vi "start.vi"(8 "error in (no error)":errorcluster, 11 "DAQmx_pulse_out in":refnum<class "DAQmx_DO.lvclass">) -> (0 "error out":errorcluster, 3 "DAQmx_pulse_out out":refnum<class "DAQmx_DO.lvclass">)   [LabVIEW 2013, in "DAQmx_DO.lvclass"]
uses:
  DAQmx_DO.lvclass
  DAQmx_DO.lvclass/DAQmx_DO.ctl
  Globals.vi
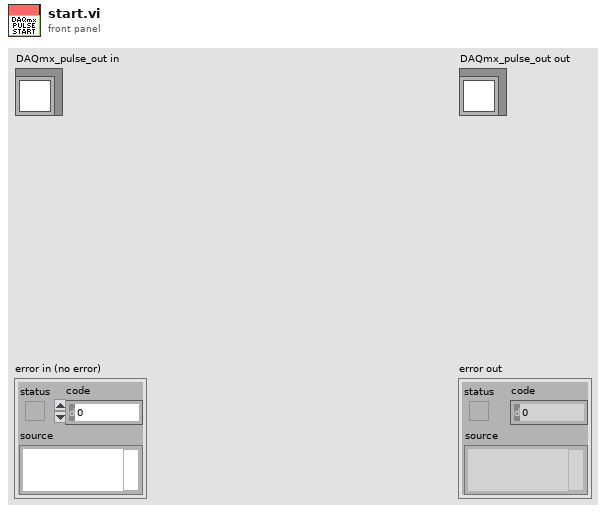
[diagram p1: front panel]
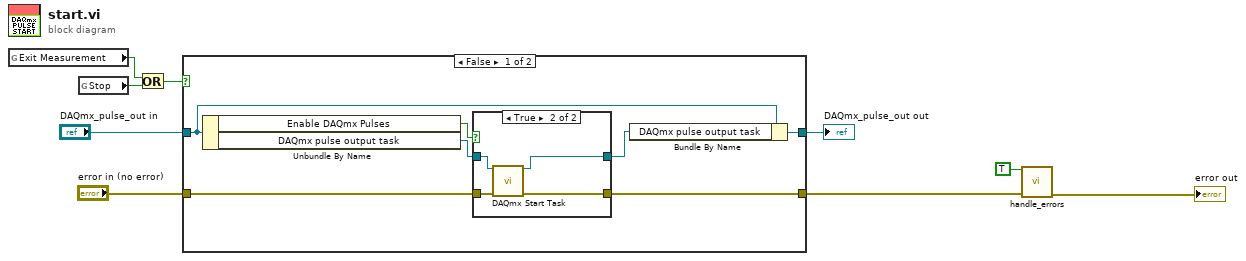
[diagram p0: block diagram]
diagram:
  n1 = global read "Globals.vi" "Exit Measurement"() -> (w6:bool)
  n2 = global read "Globals.vi" "Stop"() -> (w7:bool)
  n3 = Or(x=w6, y=w7) -> (x .or. y?=w5:bool)
  n4 = case shown="False" w5 {
    tunnel: [w11 w23] -> w2
    tunnel: [w13 w24] -> w8
    tunnel: "DAQmx_pulse_out in" -> [w14 w24]
    tunnel: "error in (no error)" -> [w10 w23]
    frame False {
      n5 = Unbundle By Name(w14) -> ("Enable DAQmx Pulses"=w16:bool, "DAQmx pulse output task"=w15:refnum<k21>)
      n6 = case shown="True" w16 {
        tunnel: w10 -> [w18 w22]
        tunnel: w15 -> [w17 w21]
        tunnel: [w18 w19] -> w11
        tunnel: [w17 w20] -> w12
        frame False {
        }
        frame True {
          n7 = call <vilib>:"DAQmx Start Task.vi"("task/channels in"=w21, "error in"=w22) -> ("task out"=w20:refnum<k21>, "error out"=w19:errorcluster)  [unwired: 12 in]
        }
      }
      n8 = Bundle By Name(cluster=w14, "DAQmx pulse output task"=w12) -> (w13:refnum<class "DAQmx_DO.lvclass">)
    }
    frame True {
    }
  }
  "DAQmx_pulse_out out" <- w8
  n9 = call "handle_errors.vi"("Exit Operation"=TRUE ("Exit Measurement"), "error in (no error)"=w2) -> ("error out"=→"error out":errorcluster)  [unwired: 13 in]
